vi "Create.vi"(8 "error in (no error)":errorcluster, 10 "Element":refnum<class "Config Element.lvclass">) -> (0 "error out":errorcluster, 3 "Node out":refnum<class "Node.lvclass">)   [LabVIEW 2020, in "VolatusConfig.lvlib" / "Node.lvclass"]
uses:
  Node.lvclass
  C:/dev/lv20CE/relink/lv-volatus/VolatusConfig/VolatusConfigElement/VolatusConfigElement.lvclass
  lv-cdm/CDM-Config/Config Element/Config Element.lvclass
  Node.lvclass/Node.ctl
  VolatusConfigElement/VolatusConfigElement.lvclass
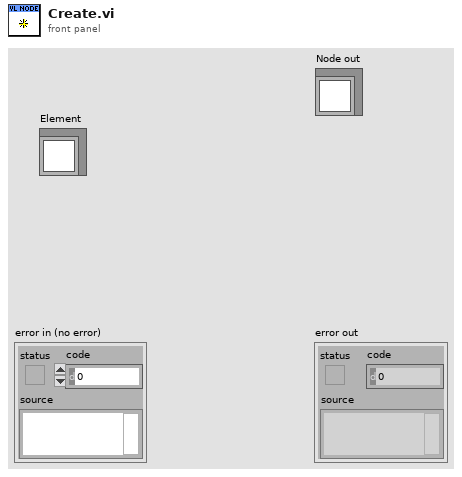
[diagram p1: front panel]
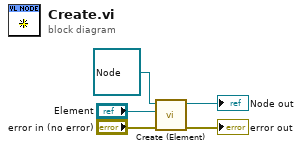
[diagram p0: block diagram]
diagram:
  n1 = call "Create (Element).vi"("error in (no error)"="error in (no error)", "Element"="Element", "VolatusConfigElement in"=refnum<class "Node.lvclass"> refnum ("Node in")) -> ("error out"=→"error out":errorcluster, "VolatusConfigElement out"=→"Node out":refnum<class "Node.lvclass">)  [unwired: 7 in]
